vi "CC Script Parse Set Outlet.vi"(8 "error in (no error)":errorcluster, 9 "To Script?":bool, 10 "outlet parm in":T1, 11 "DefineObject Parameters":string="Wheel1=3,Wheel2=5") -> (0 "error out":errorcluster, 2 "Script Out":string="ObjectName \"RA\":\"123.456\",\"DEC\":\"4546.54\"", 3 "out parm out":T1)   [LabVIEW 2024]
uses:
  typedefs/CC cluster Outlet Control.ctl
  <vilib>/regexp/Match Regular Expression.xnode
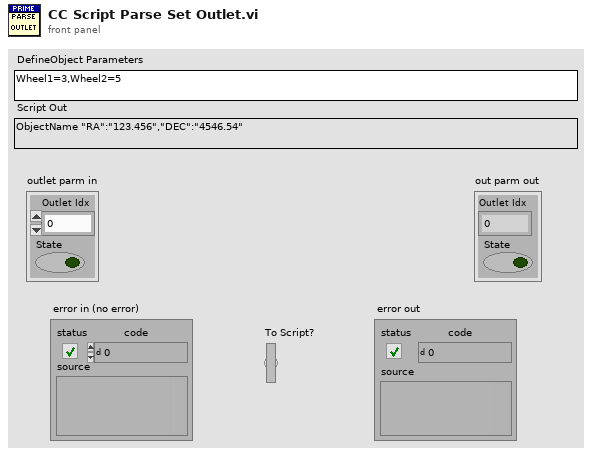
[diagram p1: front panel]
types:
  T1 = typedef "CC cluster Outlet Control.ctl" = cluster{"Outlet Idx":i32, "State":bool}
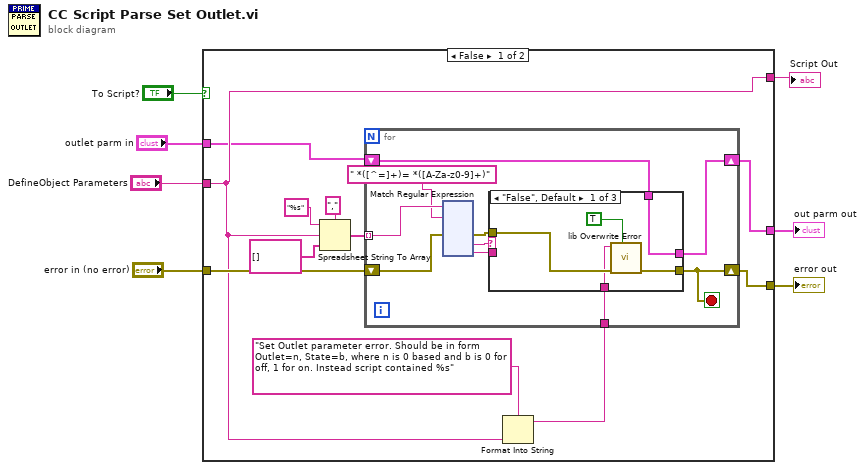
[diagram p0: block diagram]
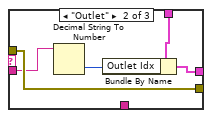
[diagram p2: hidden frame]
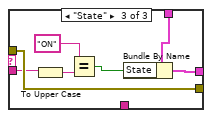
[diagram p3: hidden frame]
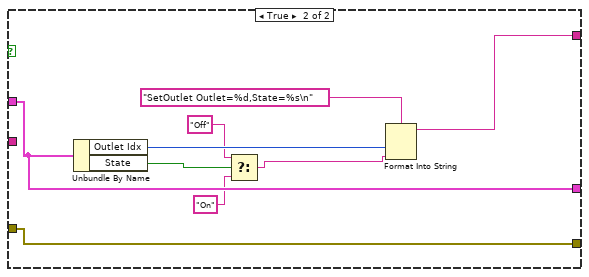
[diagram p4: hidden frame]
diagram:
  n1 = case shown="False" "To Script?" {
    tunnel: [w18 w172] -> w7
    tunnel: "error in (no error)" -> [w17 w170]
    tunnel: [w9 w170] -> w5
    tunnel: "DefineObject Parameters" -> [w12 _]
    tunnel: "outlet parm in" -> [w8 w172]
    tunnel: [w12 w171] -> w2
    frame False {
      n2 = Spreadsheet String To Array(delimiter (Tab)=",", format string="%s", spreadsheet string=w12, array type (2D Dbl)=string[] []) -> (array=w11:string[])
      n3 = Format Into String(format string="Set Outlet parameter error. Should be in form Outlet=n, State=b, where n is 0 based and b is 0 for off, 1 for on. Instead script contained %s", w12) -> (resulting string=w10:string)  [unwired: 2 in, 1 out]
      n4 = for {
        shift-right: [w27] -> w18
        shift-left: w8 -> [w28]
        tunnel: w11 -> [w26] mode=indexing
        tunnel: w10 -> [w20]
        shift-right: [w19] -> w9
        shift-left: w17 -> [w22]
        stop <- w19 stop-if-true
        n5 = xnode "Match Regular Expression"("input string"=w26, "regular expression"=" *([^=]+)= *([A-Za-z0-9]+)" ("format string"), "error in"=w22) -> ("error out"=w21:errorcluster, "submatch 1"=w24:string, "submatch 2"=w23:string)  [unwired: 3 in, 4 out]
        n6 = case shown="\"False\", Default" w24 {
          tunnel: w28 -> [w30 w38 w45]
          tunnel: [w30 w37 w44] -> w27
          tunnel: w23 -> [_ w35 w42]
          tunnel: w21 -> [w33 w36 w43]
          tunnel: w20 -> [w32 _ _]
          tunnel: [w31 w36 w43] -> w19
          frame "False", Default {
            n7 = call "lib Overwrite Error.vi"("Force Error?"=TRUE, "error in (no error)"=w33, "Error Message"=w32) -> ("error out"=w31:errorcluster)  [unwired: 8 in]
          }
          frame "Outlet" {
            n8 = Decimal String To Number(string=w35) -> (number=w34:i32)  [unwired: 2 in, 1 out]
            n9 = Bundle By Name(cluster=w38, "Outlet Idx"=w34) -> (w37:T1)
          }
          frame "State" {
            n10 = To Upper Case(1:w42) -> (0:w41:string)
            n11 = Equal?(x="ON", y=w41) -> (x = y?=w39:bool)
            n12 = Bundle By Name(cluster=w45, "State"=w39) -> (w44:T1)
          }
        }
      }
    }
    frame True {
      n13 = Unbundle By Name(w172) -> ("Outlet Idx"=w173:i32, "State"=w169:bool)
      n14 = Select(t="Off", s=w169, f="On") -> (s? t:f=w166:string)
      n15 = Format Into String(format string="SetOutlet Outlet=%d,State=%s\n", w173, w166) -> (resulting string=w171:string)  [unwired: 2 in, 1 out]
    }
  }
  "error out" <- w5
  "out parm out" <- w7
  "Script Out" <- w2
